vi "RFmxSpecAn Save Data.vi"(3 "error in (no error)":errorcluster, 4 "Harms Results":dbl[][](array[numeric])) -> (0 "error out":errorcluster)   [LabVIEW 2018]
uses:
  <vilib>/Utility/file.llb/Write Delimited Spreadsheet (DBL).vi
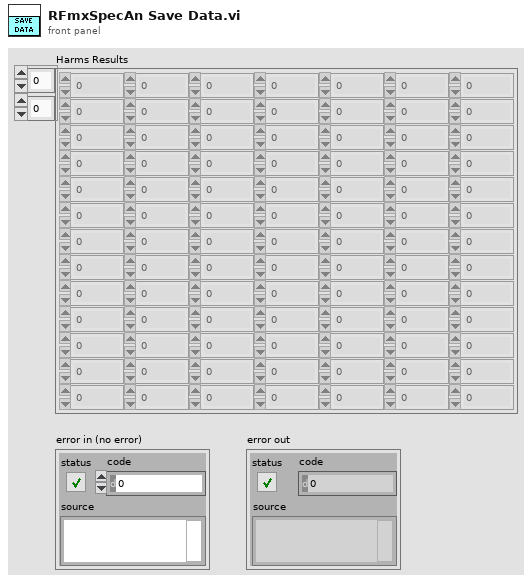
[diagram p1: front panel]
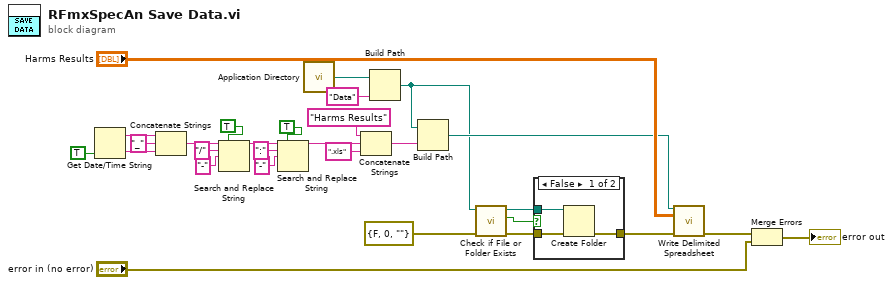
[diagram p0: block diagram]
diagram:
  n1 = Get Date/Time String(want seconds? (F)=TRUE) -> (date string=w24:string, time string=w25:string)  [unwired: 2 in]
  n2 = Concatenate Strings(w24, "_" ("string"), w25) -> (w26:string)
  n3 = Search and Replace String(replace all?=TRUE ("replace all? (F)"), input string=w26, search string="/", replace string="-" ("replace string (\"\")")) -> (result string=w27:string)  [unwired: 4 in, 3 out]
  n4 = Search and Replace String(replace all?=TRUE ("replace all? (F)"), input string=w27, search string=":", replace string="-" ("replace string (\"\")")) -> (result string=w28:string)  [unwired: 4 in, 3 out]
  n5 = call <vilib>:"Application Directory.vi"() -> ("Application Directory"=w1:path)
  n6 = Concatenate Strings("Harms Results" ("string"), w28, ".xls" ("string")) -> (w23:string)
  n7 = Build Path(base path=w1, name or relative path="Data") -> (appended path=w9:path)
  n8 = Build Path(base path=w9, name or relative path=w23) -> (appended path=w11:path)
  n9 = call <vilib>:"Check if File or Folder Exists.vi"("error in (no error)"=errorcluster {"status"=FALSE, "code"=0, "source"=""}, "path"=w9) -> ("error out"=w10:errorcluster, "file or folder exists?"=w6:bool, "dup path"=w8:path)  [unwired: 7 in]
  n10 = case shown="False" w6 {
    tunnel: w10 -> [w32 w33]
    tunnel: w8 -> [w31 _]
    tunnel: [w30 w33] -> w7
    frame False {
      n11 = Create Folder(path (use dialog)=w31, error in=w32) -> (error out=w30:errorcluster)  [unwired: 1 in, 2 out]
    }
    frame True {
    }
  }
  n12 = call-poly <vilib>:"Write Delimited Spreadsheet.vi"("file path (dialog if empty)"=w11, "2D data"="Harms Results", "error in (no error)"=w7) -> ("error out"=w4:errorcluster)  [unwired: 11 in, 1 out]
  n13 = Merge Errors(w4, "error in (no error)") -> (→"error out":errorcluster)
